vi "SVT Decimated Exp Avg Sound Level (1 Ch).vi"(6 "restart averaging (F)":bool, 7 "decimation factor":i32=-1, 8 "error in (no error)":errorcluster, 9 "time constant [ms]":dbl=125.0 format="%.2f", 10 "exponential mode":enum16{"Slow", "Fast", "Impulse", "Custom"}(ring)=enum."Fast", 11 "scaled signal [EU]":waveform(dbl)) -> (0 "error out":errorcluster, 1 "actual time constant [ms]":dbl=nan format="%.2f", 2 "unit label":string, 3 "decimated exp avg sound level [dB EU]":waveform(dbl), 5 "actual decimation factor":i32=-1)   [LabVIEW 2017]
doc: "Computes the exponential averaged sound level of <B>scaled signal [EU]</B> based on <B>exponential mode</B>, decimates this sound level by <B>decimation factor</B>, and returns the result in <B>decimated exp avg sound level [dB EU]</B>. You can use this polymorphic VI to compute the exponential averaged sound level for a single channel or for N channels. The data type you wire to the <B>scaled signal [EU]</B> input determines the polymorphic instance to use."
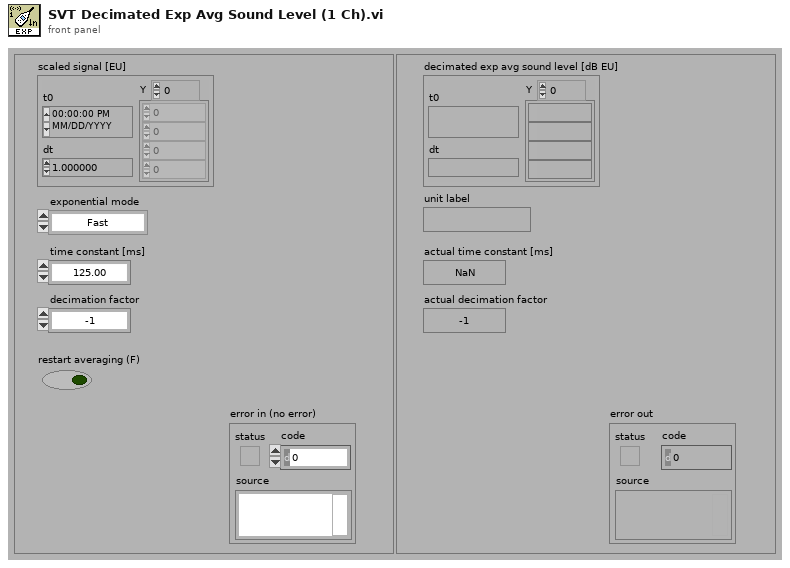
[diagram p1: front panel]
types:
  T1 = enum16{"RMS", "Running RMS", "Exp avg  ", "Dec exp avg ", "Peak", "Crest"}
  T2 = enum16{"Reset filter", "Restart averaging", "Continue processing"}
  T3 = typedef "svc_Channel Info.ctl" = cluster{"sensor sensitivity":dbl, "engineering units":T4, "dB reference":dbl, "custom label":string, "weighting filter":T5, "pregain":dbl}
  T4 = typedef "svc_Engineering Units Text Ring.ctl" = u16
  T5 = typedef "svc_Weighting Filter Text Ring.ctl" = u16
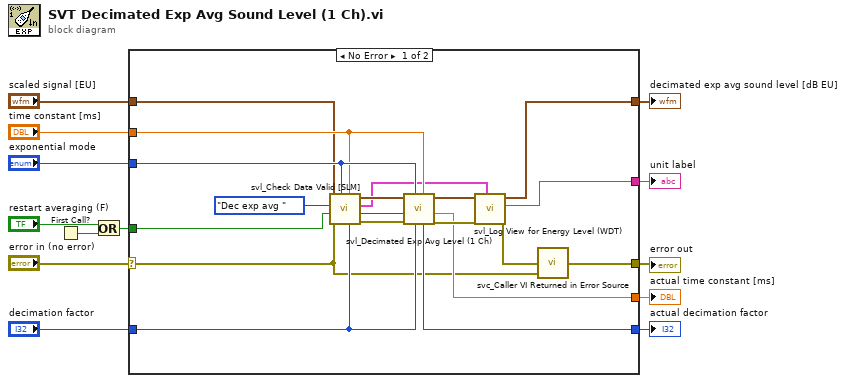
[diagram p0: block diagram]
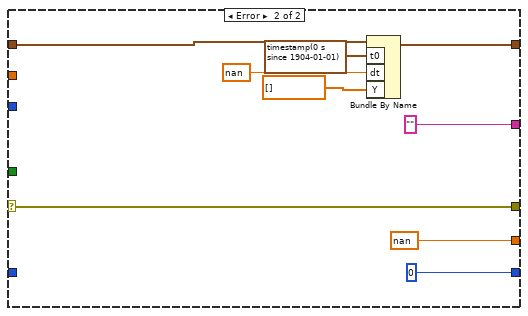
[diagram p2: hidden frame]
diagram:
  n1 = First Call?() -> (First Call?: T/F=w8:bool)
  n2 = Or(x="restart averaging (F)", y=w8) -> (x .or. y?=w7:bool)
  n3 = case shown="No Error" "error in (no error)" {
    selector: "error in (no error)" -> [w14 w41]
    tunnel: [w16 w33] -> w13
    tunnel: [w22 w41] -> w12
    tunnel: [w29 "" ("unit label")] -> w11
    tunnel: "scaled signal [EU]" -> [w15 w35]
    tunnel: w7 -> [w20 _]
    tunnel: "exponential mode" -> [w28 _]
    tunnel: "decimation factor" -> [w21 _]
    tunnel: [w27 0 ("actual decimation factor")] -> w4
    tunnel: "time constant [ms]" -> [w24 _]
    tunnel: [w23 nan ("actual time constant [ms]")] -> w2
    frame No Error {
      n4 = call <vilib>:"svl_Check Data Valid [SLM].vi"("decimation factor"=w21, "time constant [ms]"=w24, "exponential mode"=w28, "error in (no error)"=w14, "restart averaging (F)"=w20, "Level Analysis"=T1."Dec exp avg ", "scaled signal [EU]"=w15) -> ("error out"=w32:errorcluster, "processing state"=w25:T2, "channel info"=w17:T3, "dup scaled signal [EU]"=w18:waveform(dbl))  [unwired: 1 in]
      n5 = call <vilib>:"svl_Decimated Exp Avg Level (1 Ch).vi"("time constant [ms]"=w24, "decimation factor"=w21, "exponential mode"=w28, "error in (no error)"=w32, "processing state"=w25, "scaledSignal"=w18) -> ("error out"=w31:errorcluster, "actual time constant [ms]"=w23:dbl, "expAveragedArray"=w26:waveform(dbl), "actual decimation factor"=w27:i32)  [unwired: 2 in]
      n6 = call <vilib>:"svl_Log View for Energy Level (WDT).vi"("channel info"=w17, "error in (no error)"=w31, "scaledSignal"=w26) -> ("error out"=w30:errorcluster, "unit label"=w29:string, "scaledSignal"=w16:waveform(dbl))  [unwired: 6 in]
      n7 = call <vilib>:"svc_Caller VI Returned in Error Source.vi"("warning input to caller"=w14, "error in (no error)"=w30) -> ("error out"=w22:errorcluster)  [unwired: 3 in]
    }
    frame Error {
      n8 = Bundle By Name(cluster=w35, "t0"=timestamp(0 s since 1904-01-01), "dt"=nan ("t0"), "Y"=dbl[] []) -> (w33:waveform(dbl))
    }
  }
  "unit label" <- w11
  "actual time constant [ms]" <- w2
  "decimated exp avg sound level [dB EU]" <- w13
  "error out" <- w12
  "actual decimation factor" <- w4
